vi "VG_Barre_Progression_ISO_P.vi"() -> ()   [LabVIEW 2020]
panel:
  out "VG_Barre_Progression":dbl(slide) scale=0.0..100.0
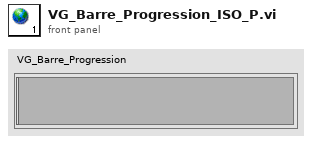
[diagram p1: front panel]
diagram:
